vi "ARC_Queue Destroy_Single.vi"(8 "error in (no error)":errorcluster caption="Error In (no error)", 11 "Queue Name(unamed)":string) -> (0 "error out":errorcluster caption="Error Out", 2 "Remaining Elements":cluster{"Event":string, "Data":variant}[](array[cluster]), 3 "Queue Name":string)   [LabVIEW 2016]
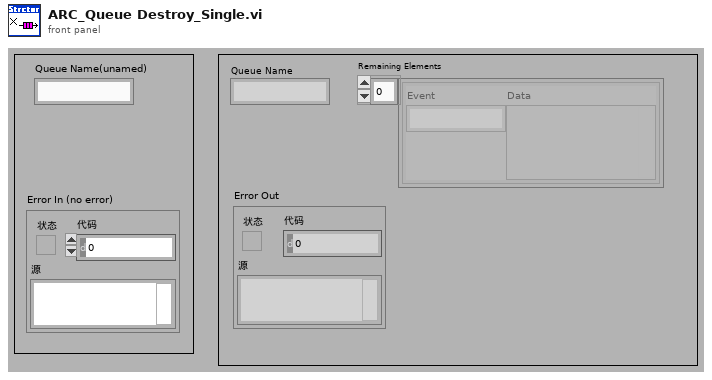
[diagram p1: front panel]
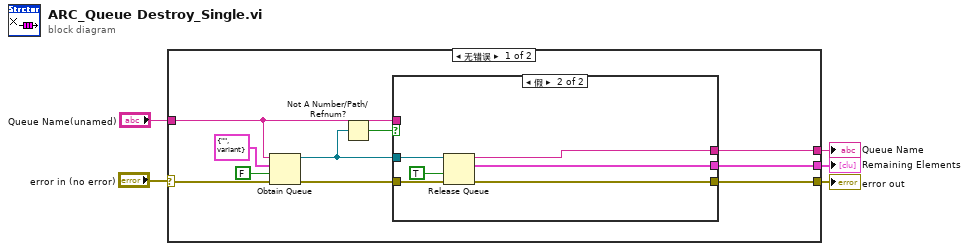
[diagram p0: block diagram]
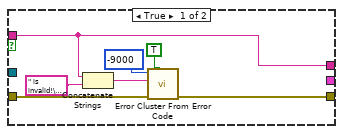
[diagram p2: hidden frame]
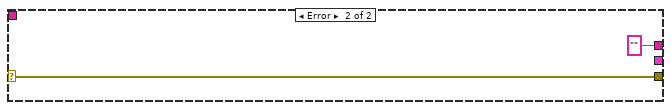
[diagram p3: hidden frame]
diagram:
  n1 = case shown="无错误" "error in (no error)" {
    selector: "error in (no error)" -> [w14 w30]
    tunnel: [w15 w30] -> w5
    tunnel: "Queue Name(unamed)" -> [w9 _]
    tunnel: [w7 _] -> w2
    tunnel: [w6 "" ("queue name")] -> w1
    frame No Error {
      n2 = Obtain Queue(name (unnamed)=w9, element data type=cluster{"Event":string, "Data":variant} {"Event"="", "Data"=variant} ("输出簇"), create if not found? (T)=FALSE ("如未找到是否创建？(T)"), error in (no error)=w14) -> (queue out=w11:refnum<queue>, error out=w10:errorcluster)  [unwired: 1 in, 1 out]
      n3 = Not A Number/Path/Refnum?(number/path/refnum=w11) -> (NaN/Path/Refnum?=w12:bool)
      n4 = case shown="假" w12 {
        tunnel: w10 -> [w18 w25]
        tunnel: [w17 w26] -> w15
        tunnel: [w19 w28] -> w6
        tunnel: [_ w27] -> w7
        tunnel: w9 -> [w19 _]
        tunnel: w11 -> [_ w23]
        frame True {
          n5 = Concatenate Strings(w19, " is invalid!\nEnsure the queue has been created!" ("字符串")) -> (w22:string)
          n6 = call <vilib>:"Error Cluster From Error Code.vi"("show call chain? (False)"=TRUE, "error in (no error)"=w18, "error message (\"\")"=w22, "error code (0)"=-9000) -> ("error out"=w17:errorcluster)  [unwired: 5 in]
        }
        frame False {
          n7 = Release Queue(queue=w23, force destroy? (F)=TRUE ("强制销毁？(F)"), error in (no error)=w25) -> (queue name=w28:string, remaining elements=w27:cluster{"Event":string, "Data":variant}[], error out=w26:errorcluster)
        }
      }
    }
    frame Error {
    }
  }
  "error out" <- w5
  "Queue Name" <- w1
  "Remaining Elements" <- w2
